vi "SmoothTool.vi"(8 "Calling VI REF":refnum<vi>, 11 "Display REFs In":refnum<vi>[](array[refnum])) -> ()   [LabVIEW 2014]
uses:
  <vilib>/Utility/cursorutil.llb/Set Cursor (Icon Pict).vi
panel:
  in  "Smooth Amount (Sigma)":dbl=1.0
  in  "Select Image":bool
  in  "Exit":bool
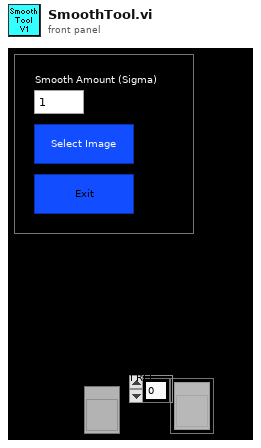
[diagram p1: front panel]
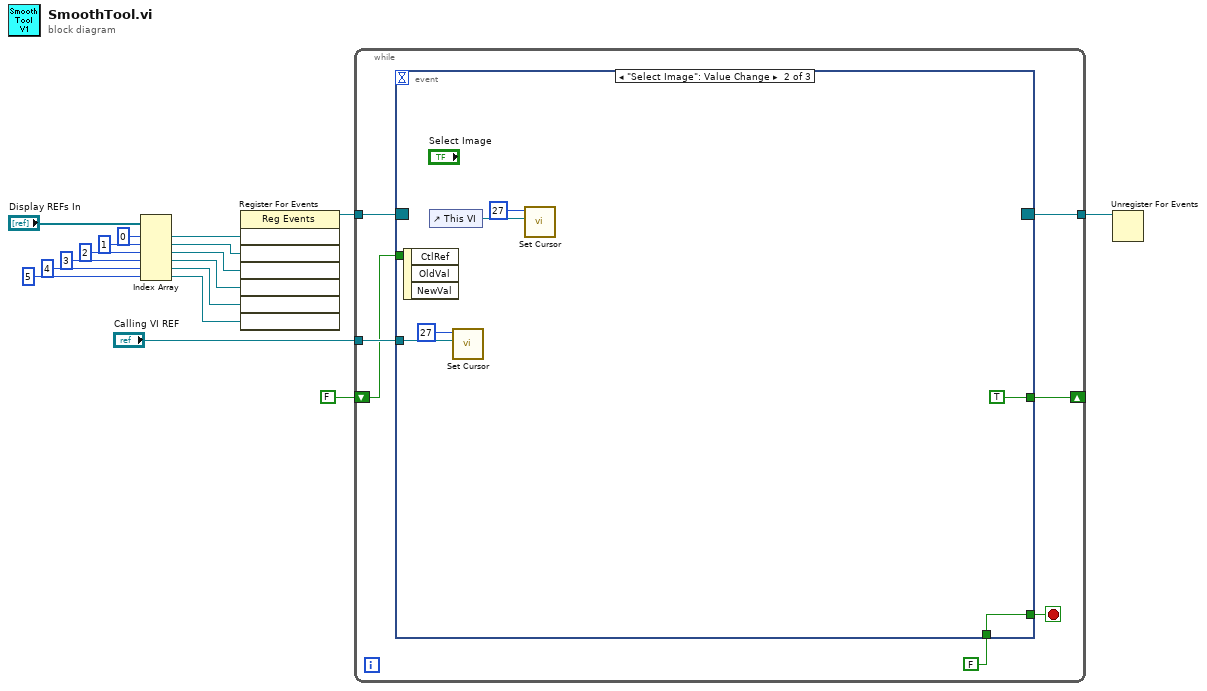
[diagram p0: block diagram]
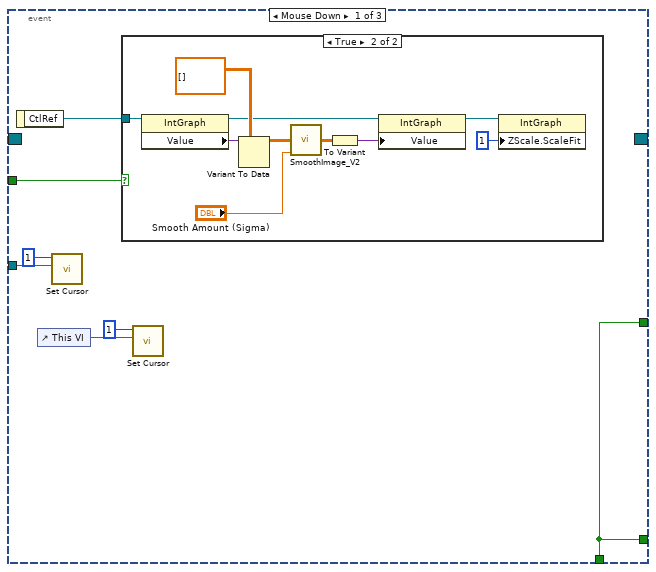
[diagram p2: hidden frame]
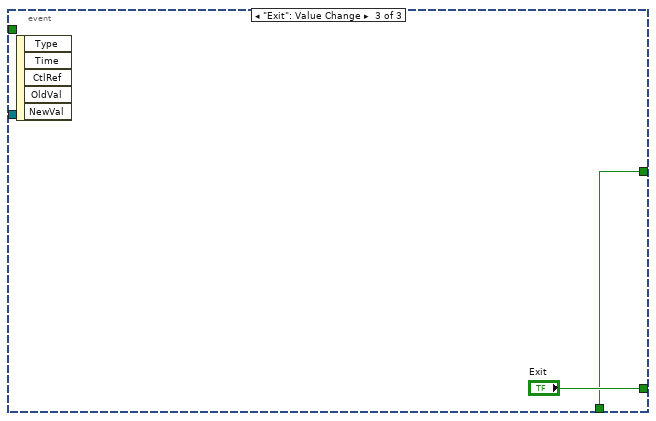
[diagram p4: hidden frame]
diagram:
  n1 = Index Array(array="Display REFs In", index #1=0 ("index"), index #2=1 ("index"), index #3=2 ("index"), index #4=3 ("index"), index #5=4 ("index"), index #6=5 ("index")) -> (element #1=w4:refnum<vi>, element #2=w7:refnum<vi>, element #3=w8:refnum<vi>, element #4=w9:refnum<vi>, element #5=w10:refnum<vi>, element #6=w11:refnum<vi>)
  n2 = register-events(w4, w7, w8, w9, w10, w11) -> (reference out=w6:refnum<event-registration>)  [unwired: 2 in, 1 out]
  n3 = while {
    tunnel: w6 -> [w22]
    tunnel: [w21] -> w5
    tunnel: "Calling VI REF" -> [w20]
    shift-right: [w19] -> _
    shift-left: FALSE -> [w18]
    stop <- w24 stop-if-true
    n4 = event shown="[1] \"Select Image\": Value Change" {
      selector: w22 -> [_ _ _]
      dyn-events: [_ _ _] -> w21
      timeout: _ -> [_ _ _]
      tunnel: [w26 w47 "Exit"] -> w24
      tunnel: FALSE -> [w26 w47 w48]
      tunnel: w20 -> [w29 w45 _]
      tunnel: [w26 TRUE w48] -> w19
      tunnel: w18 -> [w25 _ _]
      event Mouse Down {
        n5 = event-data() -> ("CtlRef"=w31:refnum<vi>)  [unwired: 1 in]
        n6 = control-ref of="This VI"() -> (w27:refnum<vi>)
        n7 = call-poly <vilib>:"Set Cursor.vi"("VI reference (current VI)"=w29, "icon"=u16 1) -> ()  [unwired: 8 in, 2 out]
        n8 = case shown="True" w25 {
          tunnel: w31 -> [_ w41]
          frame False {
          }
          frame True {
            n9 = property class="IntGraph"(reference=w41) -> (reference out=w36:refnum<vi>, "Value"=w40:variant)  [unwired: 1 in, 1 out]
            n10 = Variant To Data(type=sgl[][] [], Variant=w40) -> (data=w38:sgl[][])  [unwired: 1 in, 1 out]
            n11 = call "SmoothImage_V2.vi"("Image IN"=w38, "Sigma (Radius)"="Smooth Amount (Sigma)") -> ("Smoothed Image"=w35:sgl[][])  [unwired: 13 in]
            n12 = To Variant(anything=w35) -> (Variant=w34:variant)
            n13 = property class="IntGraph"(reference=w36, "Value"=w34) -> (reference out=w33:refnum<vi>)  [unwired: 1 in, 1 out]
            n14 = property class="IntGraph"(reference=w33, "ZScale.ScaleFit"=u8 1 ("Z Scale.Scale Fit")) -> ()  [unwired: 1 in, 2 out]
          }
        }
        n15 = call-poly <vilib>:"Set Cursor.vi"("VI reference (current VI)"=w27, "icon"=u16 1) -> ()  [unwired: 8 in, 2 out]
      }
      event "Select Image": Value Change {
        n16 = event-data() -> ()  [unwired: 1 in, 3 out]
        n17 = control-ref of="This VI"() -> (w43:refnum<vi>)
        n18 = call-poly <vilib>:"Set Cursor.vi"("VI reference (current VI)"=w45, "icon"=u16 27) -> ()  [unwired: 8 in, 2 out]
        n19 = call-poly <vilib>:"Set Cursor.vi"("VI reference (current VI)"=w43, "icon"=u16 27) -> ()  [unwired: 8 in, 2 out]
      }
      event "Exit": Value Change {
        n20 = event-data() -> ()  [unwired: 1 in, 5 out]
      }
    }
  }
  n21 = Unregister For Events(event registration refnum=w5) -> ()  [unwired: 1 in, 1 out]
